vi "MES操作函数条码1.vi"(7 "SN":string="0105442MF011400002", 8 "error in (no error)":errorcluster caption="错误输入（无错误）", 11 "MES配置":T2={"接口地址："="http://10.9.30.175:50100/manufacturing/IntegrationServlet?InterType=XML&message=", "SITE（站点）   "="A157", "PWD（口令）"="123456", "RESOURCE（资源）"="A-6-Z-TEST", "OPERATION（工序）"="Z-TEST", "USER（用户）"="TEST", "QTY"="", "ACTIVITY"="", "NC_CODE（NG代码）"="", "启用MES"=TRUE}) -> (0 "error out":errorcluster caption="错误输出", 3 "逻辑与":bool)   [LabVIEW 2011]
panel:
  out "输出簇":T1
  out "数组":string[](array[string])
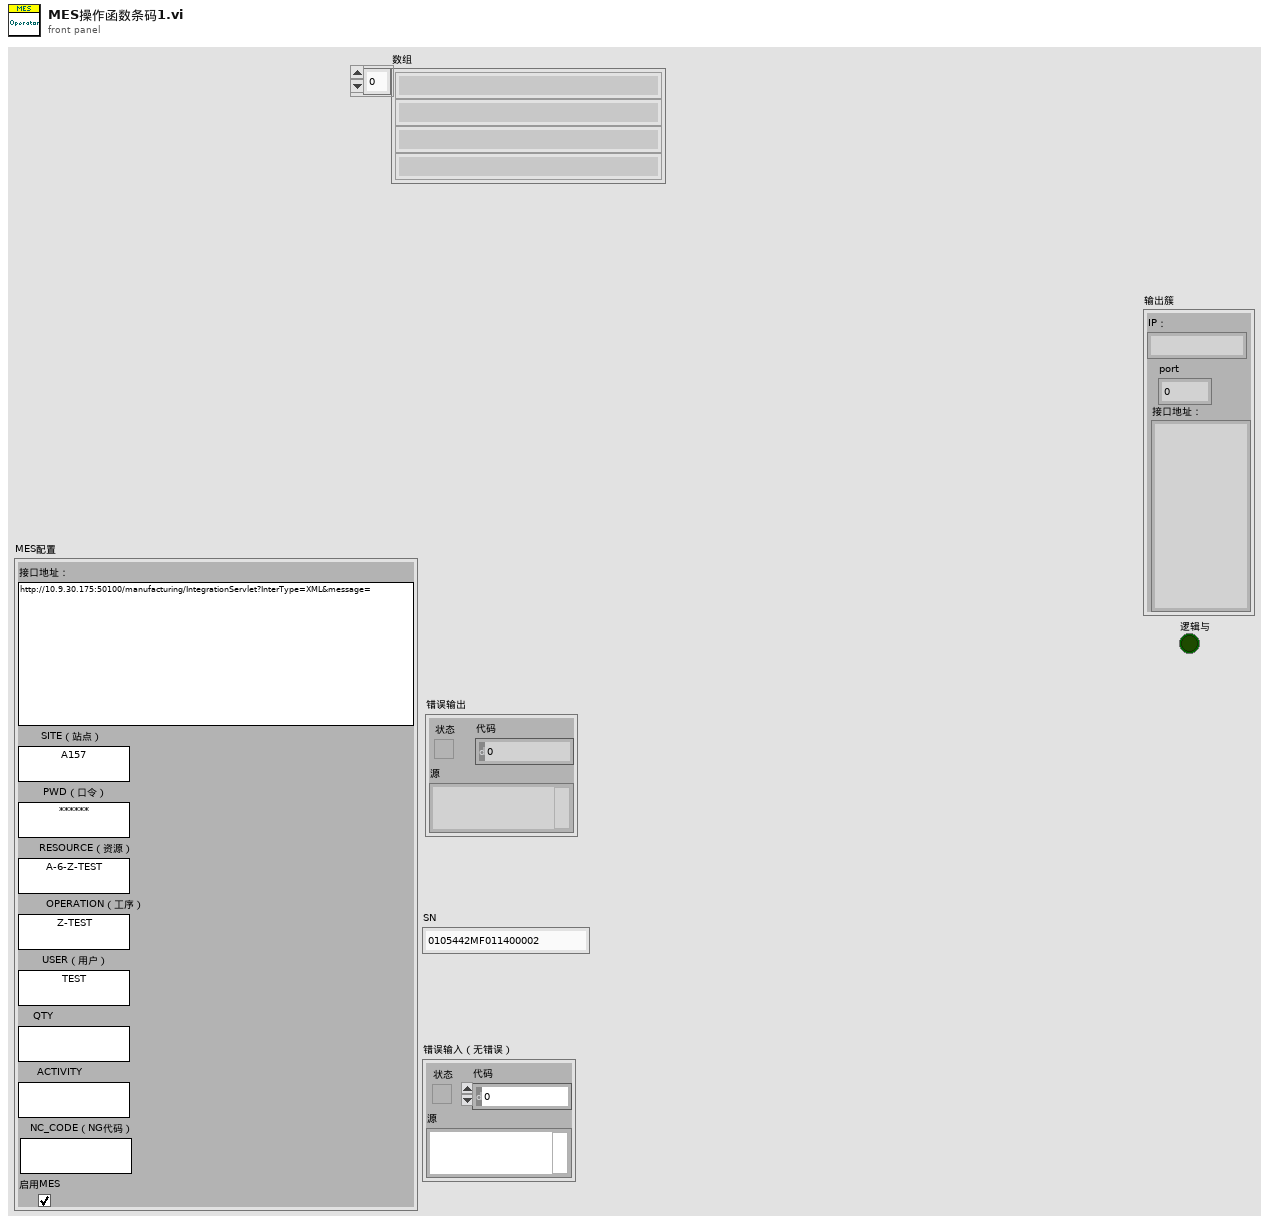
[diagram p1: front panel]
types:
  T1 = cluster{"IP：":string, "port":i32, "接口地址：":string}
  T2 = typedef "MES设置.ctl" = cluster{"接口地址：":string, "SITE（站点）   ":string, "PWD（口令）":string, "RESOURCE（资源）":string, "OPERATION（工序）":string, "USER（用户）":string, "QTY":string, "ACTIVITY":string, "NC_CODE（NG代码）":string, "启用MES":bool}
  T3 = enum16{"USER_CHECK", "SFC_CHECK", "RLT_PASS", "RLT_ERROR", "RES_AREA"}
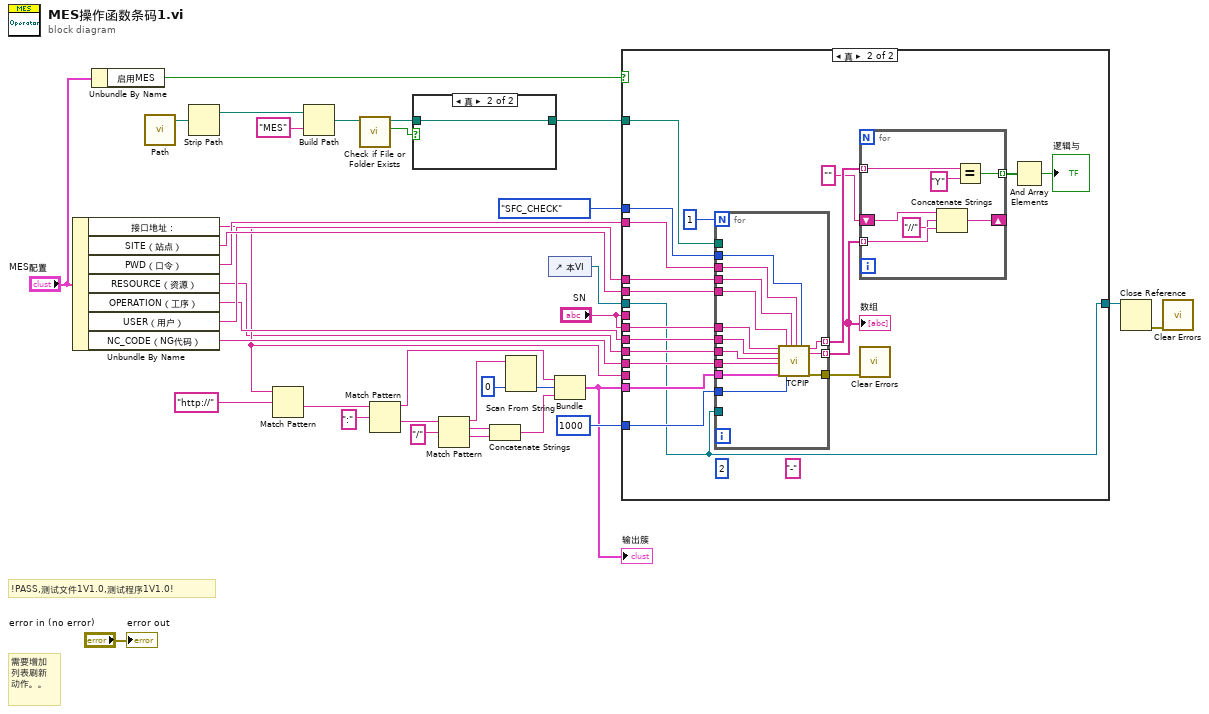
[diagram p0: block diagram]
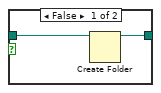
[diagram p2: hidden frame]
diagram:
  # "!PASS,测试文件1V1.0,测试程序1V1.0!"
  # "需要增加\n列表刷新\n动作。。"
  n1 = Unbundle By Name("MES配置") -> ("接口地址："=w16:string, "SITE（站点）"=w33:string, "PWD（口令）"=w31:string, "RESOURCE（资源）"=w15:string, "OPERATION（工序）"=w30:string, "USER（用户）"=w32:string, "NC_CODE（NG代码）"=w29:string)
  n2 = Unbundle By Name("MES配置") -> ("启用MES"=w4:bool)
  n3 = call "Path.vi"() -> ("appended path"=w9:path)  [unwired: 11 in]
  n4 = Strip Path(path=w9) -> (stripped path=w10:path)  [unwired: 1 out]
  n5 = Match Pattern(string=w16, regular expression="http://" ("正则表达式")) -> (after substring=w26:string)  [unwired: 1 in, 3 out]
  n6 = Build Path(base path=w10, name or relative path="MES" ("名称或相对路径")) -> (appended path=w12:path)
  n7 = call <vilib>:"Check if File or Folder Exists.vi"("path"=w12) -> ("file or folder exists?"=w13:bool, "dup path"=w14:path)  [unwired: 8 in, 1 out]
  n8 = Match Pattern(string=w26, regular expression=":" ("正则表达式")) -> (before substring=w21:string, after substring=w24:string)  [unwired: 1 in, 2 out]
  n9 = case shown="真" w13 {
    tunnel: w14 -> [w37 w39]
    tunnel: [w38 w39] -> w8
    frame False {
      n10 = Create Folder(path (use dialog)=w37) -> (created path=w38:path)  [unwired: 2 in, 2 out]
    }
    frame True {
    }
  }
  n11 = Match Pattern(string=w24, regular expression="/" ("正则表达式")) -> (before substring=w22:string, match substring=w1:string, after substring=w3:string)  [unwired: 1 in, 1 out]
  n12 = Concatenate Strings(w1, w3) -> (w2:string)
  n13 = Scan From String(input string=w22, default 1=0 ("默认值 1")) -> (output 1=w19:i32)  [unwired: 3 in, 3 out]
  n14 = control-ref of="本VI"() -> (w7:refnum<vi>)
  n15 = Bundle("接口地址："=w21, "默认值 1"=w19, w2) -> (w20:cluster{"接口地址：":string, "默认值 1":i32, string})  [unwired: 1 in]
  "输出簇" <- w20
  n16 = case shown="真" w4 {
    tunnel: T3."SFC_CHECK" ("STATE") -> [_ w59]
    tunnel: w33 -> [_ w58]
    tunnel: w32 -> [_ w57]
    tunnel: w31 -> [_ w56]
    tunnel: "SN" -> [_ w55]
    tunnel: w30 -> [_ w44]
    tunnel: w29 -> [_ w54]
    tunnel: u64 1000 ("TCP超时") -> [_ w53]
    tunnel: w20 -> [_ w52]
    tunnel: "SN" -> [_ _]
    tunnel: w16 -> [_ _]
    tunnel: w15 -> [_ w45]
    tunnel: w7 -> [w40 w42]
    tunnel: w8 -> [_ w43]
    tunnel: [w40 w42] -> w6
    frame False {
    }
    frame True {
      (unwired) 2
      (unwired) "-" ("搜索字符串")
      n17 = for {
        N: 1 -> [_]
        tunnel: w58 -> [w78]
        tunnel: w57 -> [w77]
        tunnel: w56 -> [w76]
        tunnel: w55 -> [w75]
        tunnel: w44 -> [w74]
        tunnel: w45 -> [w73]
        tunnel: w54 -> [w72]
        tunnel: w53 -> [w71]
        tunnel: w52 -> [w70]
        tunnel: [w69] -> w48 mode=indexing
        tunnel: [w68] -> w50 mode=indexing
        tunnel: [w67] -> w46
        tunnel: w43 -> [_]
        tunnel: w42 -> [_]
        tunnel: w59 -> [w79]
        n18 = call "TCPIP.vi"("SFC"=w75, "OPERATOR"=w74, "RESOURCE"=w73, "NC_CODE"=w72, "SERVER"=w70, "SITE"=w78, "TCP超时"=w71, "USER"=w77, "PWD"=w76, "STATE"=w79) -> ("Y&N"=w68:string, "系统消息"=w69:string, "error out"=w67:errorcluster)  [unwired: 7 in]
      }
      "数组" <- w48
      n19 = for {
        tunnel: w50 -> [w66] mode=indexing
        tunnel: [w64] -> w49 mode=indexing
        tunnel: w48 -> [w63] mode=indexing
        shift-right: [w62] -> _
        shift-left: "" -> [w61]
        n20 = Concatenate Strings(w61, "//" ("字符串"), w63) -> (w62:string)
        n21 = Equal?(x=w66, y="Y") -> (x = y?=w64:bool)
      }
      n22 = call <vilib>:"Clear Errors.vi"("error in (no error)"=w46) -> ()  [unwired: 6 in, 1 out]
      n23 = And Array Elements(Boolean array=w49) -> (logical AND=→"逻辑与":bool)
    }
  }
  n24 = Close Reference(reference=w6) -> (error out=w5:errorcluster)  [unwired: 1 in]
  n25 = call <vilib>:"Clear Errors.vi"("error in (no error)"=w5) -> ()  [unwired: 6 in, 1 out]
  "error out" <- "error in (no error)"
